vi "test_Loop OpenClose (lowLevel).vi"() -> ()   [LabVIEW 2020]
uses:
  <instrlib>/AIM GmbH/_AIM 664/AIM664LV.lvlib
  <instrlib>/AIM GmbH/_AIM 664/bsp/Fdx Create Session (Tx-UDP Port-Oriented).vi
panel:
  in  "simulate execution time mS":u32=100
  in  "idle before iterations mS":u32=1000
  out "error out":errorcluster
  out "executed":i32
  in  "Iterations":i32=1
  out "instances count 2":i32
  out "instances count":i32
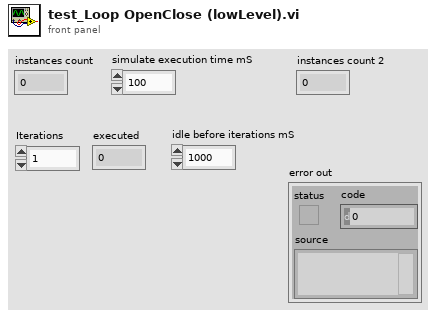
[diagram p1: front panel]
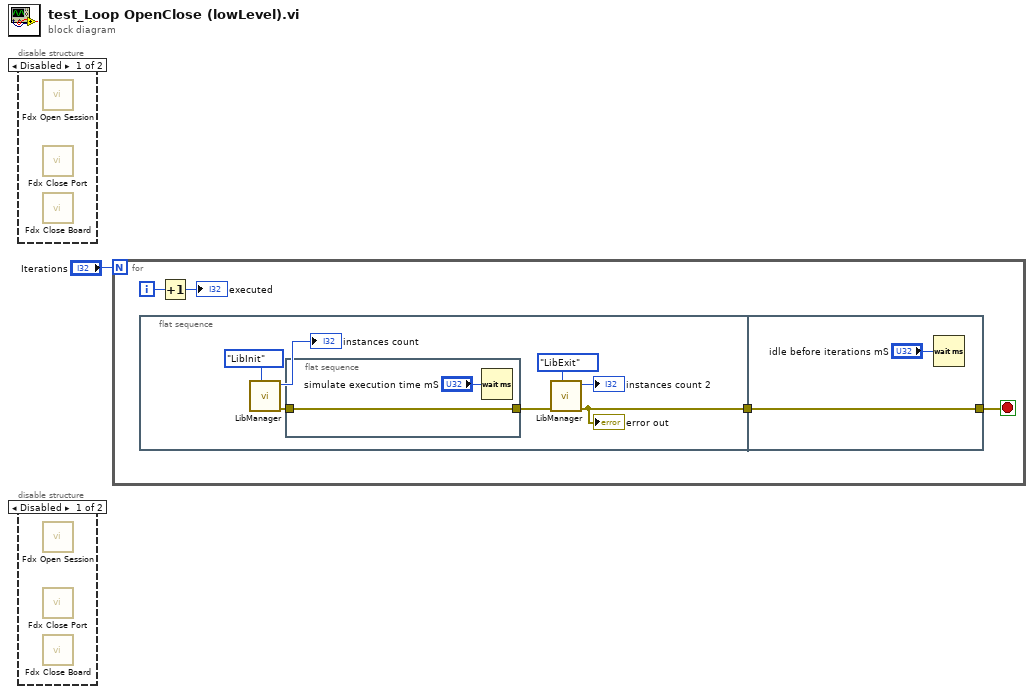
[diagram p0: block diagram]
diagram:
  n1 = disable-structure shown="Disabled" {
    frame Disabled {
      n2 = call-poly <instrlib>:"Fdx Open Session.vi"() -> ()  [unwired: 7 in, 5 out]
      n3 = call <instrlib>:"Fdx Close Port.vi"() -> ()  [unwired: 10 in, 2 out]
      n4 = call <instrlib>:"Fdx Close Board.vi"() -> ()  [unwired: 11 in, 1 out]
    }
    frame Enabled {
    }
  }
  n5 = disable-structure shown="Disabled" {
    frame Disabled {
      n6 = call-poly <instrlib>:"Fdx Open Session.vi"() -> ()  [unwired: 7 in, 5 out]
      n7 = call <instrlib>:"Fdx Close Port.vi"() -> ()  [unwired: 10 in, 2 out]
      n8 = call <instrlib>:"Fdx Close Board.vi"() -> ()  [unwired: 11 in, 1 out]
    }
    frame Enabled {
    }
  }
  n9 = for {
    N: "Iterations" -> [_]
    i -> [w3]
    stop <- w5 stop-if-true
    n10 = flat-sequence {
      tunnel: [w8] -> w4
      tunnel: [w15] -> w5
      tunnel: w4 -> [w15]
      frame #0 {
        n11 = call <instrlib>:"LibManager.vi"("action"=enum16{"LibInit", "LibExit"}."LibInit") -> ("error out"=w7:errorcluster, "instances count"=→"instances count":i32)  [unwired: 8 in, 1 out]
        n12 = flat-sequence {
          tunnel: w7 -> [w14]
          tunnel: [w14] -> w6
          frame #0 {
            n13 = Wait (ms)(milliseconds to wait="simulate execution time mS") -> ()  [unwired: 1 out]
          }
        }
        n14 = call <instrlib>:"LibManager.vi"("action"=enum16{"LibInit", "LibExit"}."LibExit", "error in (no error)"=w6) -> ("error out"=w8:errorcluster, "instances count"=→"instances count 2":i32)  [unwired: 7 in, 1 out]
        "error out" <- w8
      }
      frame #1 {
        n15 = Wait (ms)(milliseconds to wait="idle before iterations mS") -> ()  [unwired: 1 out]
      }
    }
    n16 = Increment(x=w3) -> (x+1=→"executed":i32)
  }
